vi "Init.vi"(7 "VolatusAPI":refnum<class "VolatusAPI.lvclass">, 8 "error in (no error)":errorcluster, 10 "Inhibit Channel":string, 11 "Element Inhibit in":refnum<class "Element Inhibit.lvclass">) -> (0 "error out":errorcluster, 3 "Element Inhibit out":refnum<class "Element Inhibit.lvclass">)   [LabVIEW 2020, in "VolatusGUI.lvlib" / "Element Inhibit.lvclass"]
uses:
  Element Inhibit.lvclass
  Volatus/VolatusAPI/VolatusAPI.lvclass
  Element Inhibit.lvclass/Element Inhibit.ctl
  lv-vecto/Vecto/Group DBL/Group DBL.lvclass
  C:/dev/lv20CE/relink/lv-vecto/Vecto/Group/Group.lvclass
  C:/dev/lv20CE/relink/lv-vecto/Vecto/Group DBL/Group DBL.lvclass
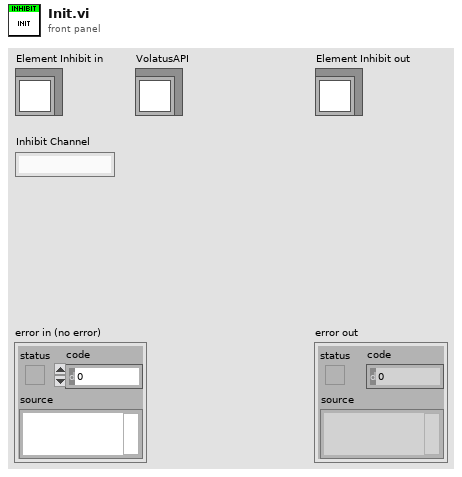
[diagram p1: front panel]
types:
  T1 = typedef "VectoConfig.lvlib/Channel Info.ctl" = cluster{"Name":string, "Group":string, "Owning Node":string, "Owning Task":string, "Resource":string}
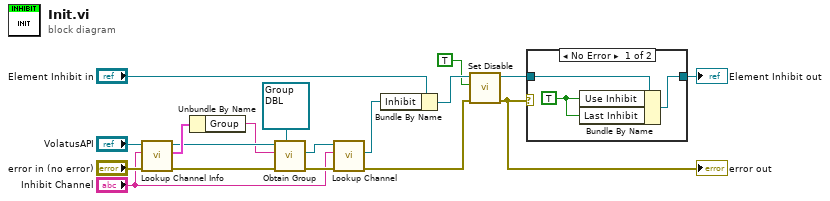
[diagram p0: block diagram]
diagram:
  n1 = call "Lookup Channel Info.vi"("error in (no error)"="error in (no error)", "Channel Name"="Inhibit Channel", "VolatusAPI in"="VolatusAPI") -> ("error out"=w10:errorcluster, "Channel Info"=w12:T1, "VolatusAPI out"=w8:refnum<class "VolatusAPI.lvclass">)  [unwired: 5 in, 1 out]
  n2 = Unbundle By Name(w12) -> ("Group"=w7:string)
  n3 = call "Obtain Group.vi"("Group Type (Abstract)"=refnum<class "Group DBL.lvclass"> refnum ("Vecto.lvlib:Group.lvclass"), "error in (no error)"=w10, "Group Name"=w7, "VolatusAPI in"=w8) -> ("error out"=w6:errorcluster, "Group"=w4:refnum<class "Group DBL.lvclass">)  [unwired: 5 in, 1 out]
  n4 = call "Lookup Channel.vi"("error in (no error)"=w6, "Channel Name"="Inhibit Channel", "Group in"=w4) -> ("error out"=w2:errorcluster, "Channel"=w3:refnum<class "Channel DBL.lvclass">)  [unwired: 6 in, 1 out]
  n5 = Bundle By Name(cluster="Element Inhibit in", "Inhibit"=w3) -> (w17:refnum<class "Element Inhibit.lvclass">)
  n6 = call "Set Disable.vi"("error in (no error)"=w2, "Disabled"=TRUE, "Element Inhibit in"=w17) -> ("error out"=w15:errorcluster, "Element Inhibit out"=w14:refnum<class "Element Inhibit.lvclass">)  [unwired: 7 in]
  "error out" <- w15
  n7 = case shown="No Error" w15 {
    tunnel: w14 -> [w21 w22]
    tunnel: [w20 w22] -> w13
    frame No Error {
      w19 = TRUE ("Use Inhibit")
      n8 = Bundle By Name(cluster=w21, "Use Inhibit"=w19, "Last Inhibit"=w19) -> (w20:refnum<class "Element Inhibit.lvclass">)
    }
    frame Error {
    }
  }
  "Element Inhibit out" <- w13
